vi "JSON to Cluster - QD.vi"(6 "Variant in":variant, 7 "Shift Pressed?":bool, 8 "error in (no error)":errorcluster, 10 "QD Combo Box Ref":refnum<vi>, 11 "QD Launch VI Ref":refnum<vi>) -> (0 "error out":errorcluster, 4 "Variant out":variant)   [LabVIEW 2013]
doc: "PLUGIN_DESCRIPTION: \nTakes the JSON text from a selected string control, and creates a cluster that can be used with the JSON functions.\nPLUGIN_DEFAULT_SHORTCUT: J"
panel:
  in  "Undo Name":string="Quick Drop Keyboard Shortcut"
  # "Do not change the connector pane of this VI.\n\nSee the block diagram for directions on how to use this template."
  # "Specify the name of the Undo transaction"
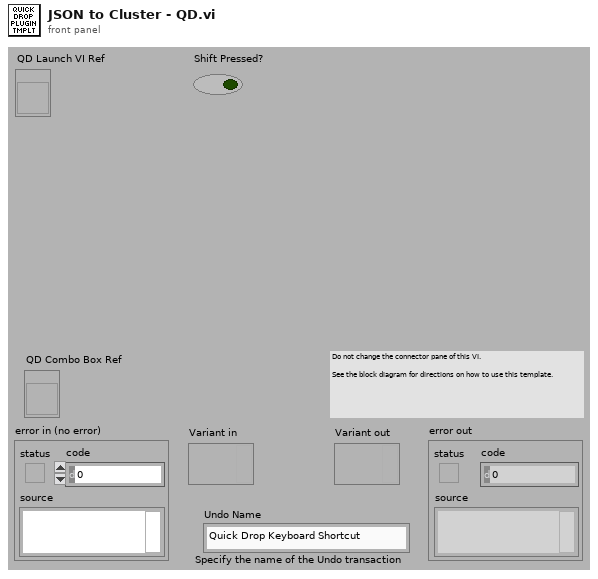
[diagram p1: front panel]
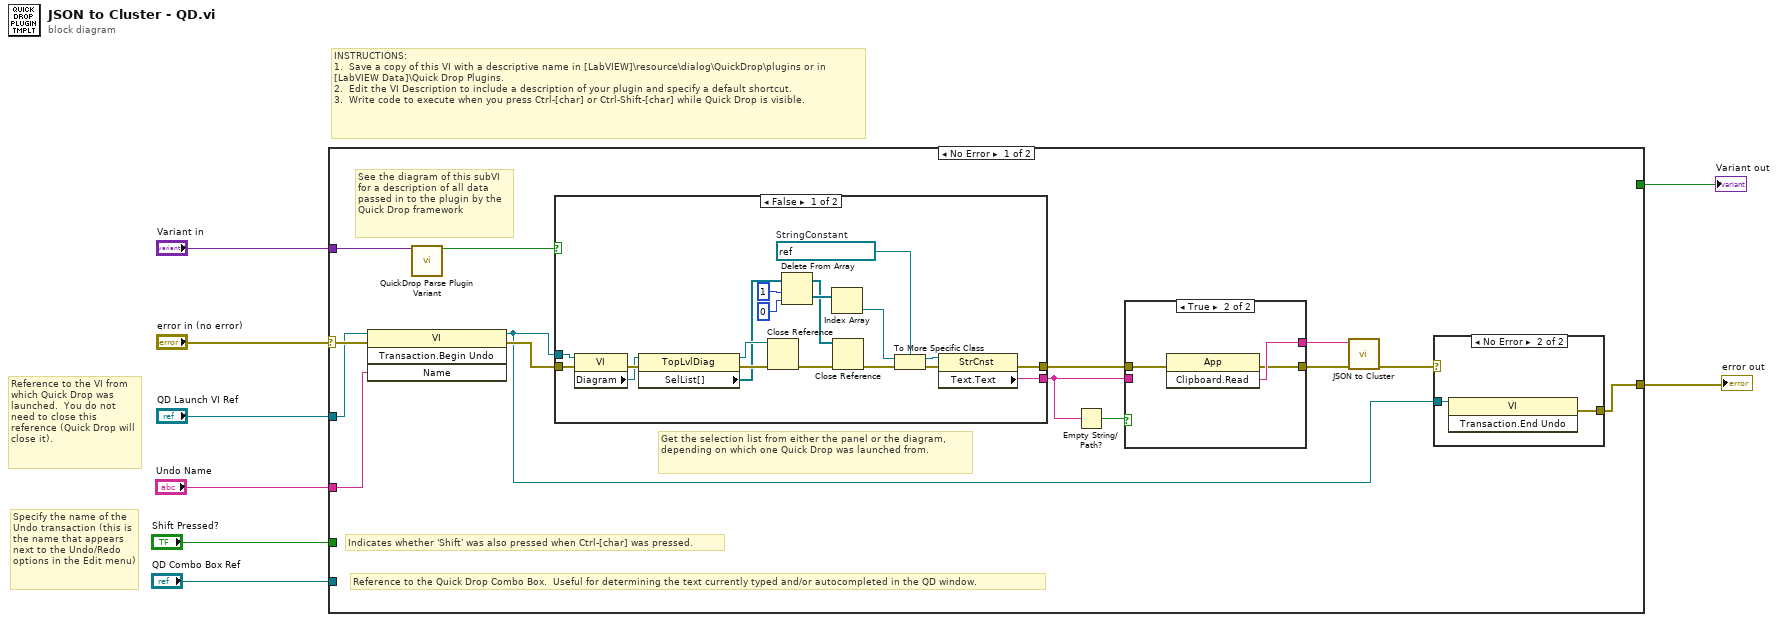
[diagram p0: block diagram]
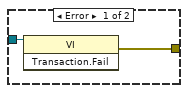
[diagram p3: hidden frame]
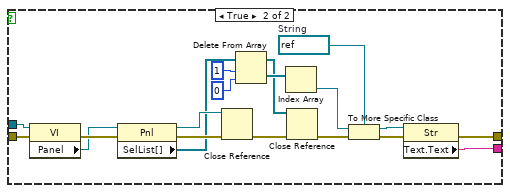
[diagram p4: hidden frame]
diagram:
  # "Specify the name of the Undo transaction (this is the name that appears next to the Undo/Redo options in the Edit menu)"
  # "Reference to the VI from which Quick Drop was launched.  You do not need to close this reference (Quick Drop will close it)."
  # "INSTRUCTIONS:\n1.  Save a copy of this VI with a descriptive name in [LabVIEW]\\resource\\dialog\\QuickDrop\\plugins or in [LabVIEW Data]\\Quick Drop Plugins.\n2.  Edit the VI Description to include a description of your plugin and specify a default shortcut. \n3.  Write code to execute when you press Ctrl-[char] or Ctrl-Shift-[char] while Quick Drop is visible."
  n1 = case shown="No Error" "error in (no error)" {
    selector: "error in (no error)" -> [w22 w71]
    tunnel: [w16 w71] -> w7
    tunnel: "QD Launch VI Ref" -> [w17 _]
    tunnel: "Shift Pressed?" -> [_ _]
    tunnel: "QD Combo Box Ref" -> [_ _]
    tunnel: "Variant in" -> [w23 _]
    tunnel: "Undo Name" -> [w21 _]
    tunnel: [TRUE _] -> w1
    frame No Error {
      # "See the diagram of this subVI for a description of all data passed in to the plugin by the Quick Drop framework"
      # "Get the selection list from either the panel or the diagram, depending on which one Quick Drop was launched from."
      # "Reference to the Quick Drop Combo Box.  Useful for determining the text currently typed and/or autocompleted in the QD window."
      # "Indicates whether 'Shift' was also pressed when Ctrl-[char] was pressed."
      n2 = invoke class="VI" method="Transaction.Begin Undo"(reference=w17, error in=w22, "Name"=w21) -> (reference out=w9:refnum<vi>, error out=w18:errorcluster)  [unwired: 1 in, 2 out]
      n3 = call <vilib>:"QuickDrop Parse Plugin Variant.vi"("QDKS Variant in"=w23) -> ("QD Launch VI Panel?"=w19:bool)  [unwired: 12 in, 2 out]
      n4 = case shown="False" w19 {
        tunnel: w18 -> [w51 w70]
        tunnel: w9 -> [w50 w69]
        tunnel: [w34 w53] -> w13
        tunnel: [w33 w52] -> w10
        frame False {
          w38 = refnum<vi> refnum  # StringConstant
          n5 = property class="VI"(reference=w50, error in=w51) -> (error out=w49:errorcluster, "Diagram"=w48:refnum<vi>)  [unwired: 1 out]
          n6 = property class="TopLvlDiag"(reference=w48, error in=w49) -> (reference out=w46:refnum<vi>, error out=w47:errorcluster, "SelList[]"=w36:refnum<vi>[])
          n7 = Close Reference(reference=w46, error in (no error)=w47) -> (error out=w35:errorcluster)
          n8 = Delete From Array(array=w36, length=1 ("longueur"), index=0 ("indice")) -> (deleted portion=w45:refnum<vi>[], array with subset deleted=w42:refnum<vi>[])
          n9 = Index Array(array=w45) -> (element=w41:refnum<vi>)  [unwired: 1 in]
          n10 = Close Reference(reference=w42, error in (no error)=w35) -> (error out=w39:errorcluster)
          n11 = To More Specific Class(target class=w38, reference=w41, error in=w39) -> (specific class reference=w40:refnum<vi>, error out=w37:errorcluster)
          n12 = property class="StrCnst"(reference=w40, error in=w37) -> (error out=w34:errorcluster, "Text.Text"=w33:string)  [unwired: 1 out]
        }
        frame True {
          w57 = refnum<vi> refnum  # String
          n13 = property class="VI"(reference=w69, error in=w70) -> (error out=w68:errorcluster, "Panel"=w67:refnum<vi>)  [unwired: 1 out]
          n14 = property class="Pnl"(reference=w67, error in=w68) -> (reference out=w65:refnum<vi>, error out=w66:errorcluster, "SelList[]"=w55:refnum<vi>[])
          n15 = Close Reference(reference=w65, error in (no error)=w66) -> (error out=w54:errorcluster)
          n16 = Delete From Array(array=w55, length=1 ("longueur"), index=0 ("indice")) -> (deleted portion=w64:refnum<vi>[], array with subset deleted=w61:refnum<vi>[])
          n17 = Index Array(array=w64) -> (element=w60:refnum<vi>)  [unwired: 1 in]
          n18 = Close Reference(reference=w61, error in (no error)=w54) -> (error out=w58:errorcluster)
          n19 = To More Specific Class(target class=w57, reference=w60, error in=w58) -> (specific class reference=w59:refnum<vi>, error out=w56:errorcluster)
          n20 = property class="Str"(reference=w59, error in=w56) -> (error out=w53:errorcluster, "Text.Text"=w52:string)  [unwired: 1 out]
        }
      }
      n21 = Empty String/Path?(string/path=w10) -> (empty?=w14:bool)
      n22 = case shown="True" w14 {
        tunnel: w13 -> [w25 w28]
        tunnel: [w24 w27] -> w12
        tunnel: [w25 w26] -> w11
        tunnel: w10 -> [w24 _]
        frame False {
        }
        frame True {
          n23 = invoke class="App" method="Clipboard.Read"(error in=w28) -> (error out=w26:errorcluster, "Read Clipbrd"=w27:string)  [unwired: 2 in, 1 out]
        }
      }
      n24 = call "JSON to Cluster.vi"("error in"=w11, "JSON String"=w12) -> ("error out"=w15:errorcluster)  [unwired: 9 in]
      n25 = case shown="No Error" w15 {
        tunnel: w9 -> [w29 w31]
        tunnel: [w30 w32] -> w16
        frame Error {
          n26 = invoke class="VI" method="Transaction.Fail"(reference=w29) -> (error out=w30:errorcluster)  [unwired: 2 in, 2 out]
        }
        frame No Error {
          n27 = invoke class="VI" method="Transaction.End Undo"(reference=w31) -> (error out=w32:errorcluster)  [unwired: 2 in, 2 out]
        }
      }
    }
    frame Error {
    }
  }
  "error out" <- w7
  "Variant out" <- w1
